vi "Generate Clamped Knot Vector.vi"(8 "error in":errorcluster, 10 "num pts":u16, 11 "degree":u16) -> (0 "error out":errorcluster, 3 "knots":u32[](array[numeric]))   [LabVIEW 2019]
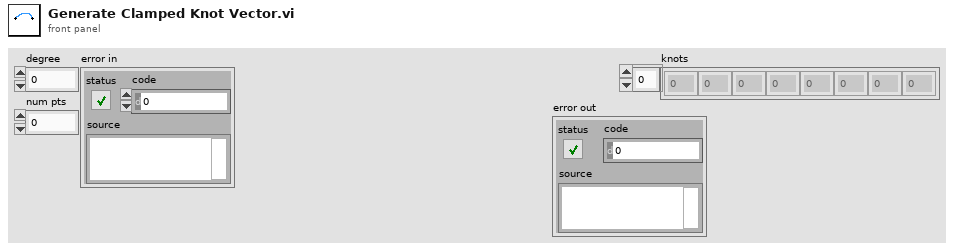
[diagram p1: front panel]
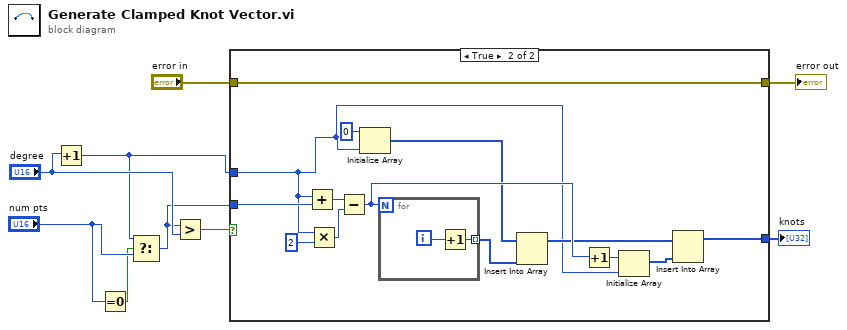
[diagram p0: block diagram]
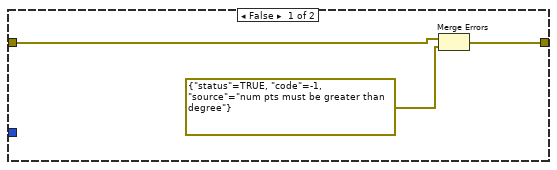
[diagram p2: hidden frame]
diagram:
  n1 = Increment(x="degree") -> (x+1=w1:u16)
  n2 = Equal To 0?(x="num pts") -> (x = 0?=w3:bool)
  n3 = Select(t=w1, s=w3, f="num pts") -> (s? t:f=w2:u16)
  n4 = Greater?(x=w2, y="degree") -> (0:w9:bool)
  n5 = case shown="True" w9 {
    tunnel: w1 -> [_ w13]
    tunnel: w2 -> [_ w26]
    tunnel: [_ w16] -> w8
    tunnel: [w12 w14] -> w6
    tunnel: "error in" -> [w10 w14]
    frame False {
      n6 = Merge Errors(w10, errorcluster {"status"=TRUE, "code"=-1, "source"="num pts must be greater than degree"} ("error constant")) -> (w12:errorcluster)
    }
    frame True {
      n7 = Add(x=w13, y=w26) -> (x+y=w25:u16)
      n8 = Multiply(x=w13, y=u32 2) -> (x*y=w23:u32)
      n9 = Subtract(x=w25, y=w23) -> (x-y=w22:u32)
      n10 = Initialize Array(0 ("dimension size"), w13) -> (w20:i32[])
      n11 = for {
        N: w22 -> [_]
        tunnel: [w27] -> w19 mode=indexing
        i -> [w28]
        n12 = Increment(x=w28) -> (x+1=w27:i32)
      }
      n13 = Insert Into Array(array=w20, new element=w19) -> (w17:i32[])  [unwired: 1 in]
      n14 = Increment(x=w22) -> (x+1=w21:u32)
      n15 = Initialize Array(w21, w13) -> (w18:u32[])
      n16 = Insert Into Array(array=w17, new element=w18) -> (w16:i32[])  [unwired: 1 in]
    }
  }
  "knots" <- w8
  "error out" <- w6
